vi "GetCustomDeviceRTDriverVIs.vi"(8 "error in (no error)":errorcluster, 11 "custom device reference in":refnum<k24>) -> (0 "error out":errorcluster, 2 "RT driver VIs":T1(array[cluster]), 3 "custom device reference out":refnum<k24>)   [LabVIEW 2016, in "VeriStandTestUtilities.lvlib"]
uses:
  VeriStandTestUtilities.lvlib
  NationalInstruments.VeriStand.XMLReader
  <vilib>/NI Veristand/Custom Device API/Custom Device Execution Mode.ctl
  <vilib>/NI VeriStand/Custom Device API/Custom Device API.lvlib
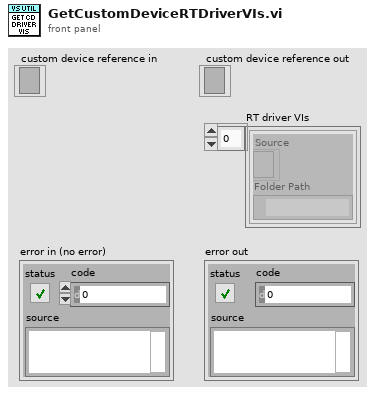
[diagram p1: front panel]
types:
  T1 = cluster{"Source":refnum<k24>, "Folder Path":path}[]
  T2 = typedef "Custom Device API.lvlib/Custom Device Execution Mode.ctl" = enum16{"Asynchronous", "Inline HW Interface", "Inline Model Interface", "Inline Timing and Sync", "Asynchronous Timing and Sync"}
  T3 = cluster{"Source":refnum<k24>, "Folder Path":path}
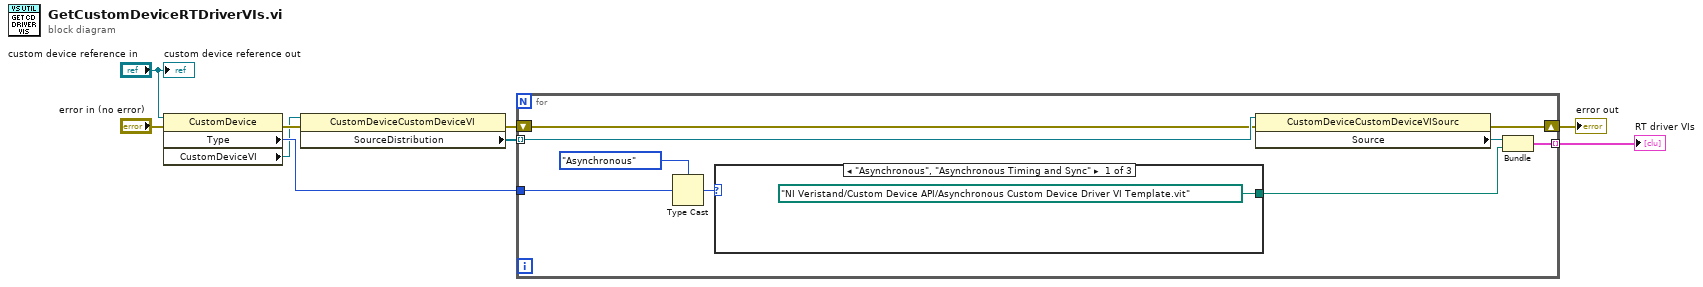
[diagram p0: block diagram]
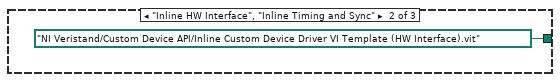
[diagram p2: hidden frame]
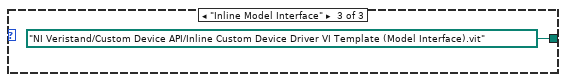
[diagram p3: hidden frame]
diagram:
  n1 = property class="CustomDevice"(reference="custom device reference in", error in="error in (no error)") -> (error out=w9:errorcluster, "Type"=w4:i32, "CustomDeviceVI"=w2:refnum<k24>)  [unwired: 1 out]
  n2 = property class="CustomDeviceCustomDeviceVI"(reference=w2, error in=w9) -> (error out=w6:errorcluster, "SourceDistribution"=w3:refnum<k24>[])  [unwired: 1 out]
  n3 = for {
    tunnel: w3 -> [w18] mode=indexing
    tunnel: [w16] -> w7 mode=indexing
    tunnel: w4 -> [w13]
    shift-right: [w11] -> w5
    shift-left: w6 -> [w10]
    n4 = Type Cast(type=Custom_Device_Execution_Mode."Asynchronous" ("Execution Mode"), x=w13) -> (*(type *) &x=w15:T2)
    n5 = case shown="\"Asynchronous\", \"Asynchronous Timing and Sync\"" w15 {
      tunnel: [path "NI Veristand/Custom Device API/Asynchronous Custom Device Driver VI Template.vit" ("Folder Path") path "NI Veristand/Custom Device API/Inline Custom Device Driver VI Template (HW Interface).vit" ("Folder Path") path "NI Veristand/Custom Device API/Inline Custom Device Driver VI Template (Model Interface).vit" ("Folder Path")] -> w12
      frame "Asynchronous", "Asynchronous Timing and Sync" {
      }
      frame "Inline HW Interface", "Inline Timing and Sync" {
      }
      frame "Inline Model Interface" {
      }
    }
    n6 = property class="CustomDeviceCustomDeviceVISourc"(reference=w18, error in=w10) -> (error out=w11:errorcluster, "Source"=w17:refnum<k24>)  [unwired: 1 out]
    n7 = Bundle("Source"=w17, "Folder Path"=w12) -> (w16:T3)  [unwired: 1 in]
  }
  "RT driver VIs" <- w7
  "error out" <- w5
  "custom device reference out" <- "custom device reference in"
